vi "电感电阻.vi"() -> ()   [LabVIEW 2017]
panel:
  out "电阻":dbl[](graph)
  out "电感":dbl[](graph)
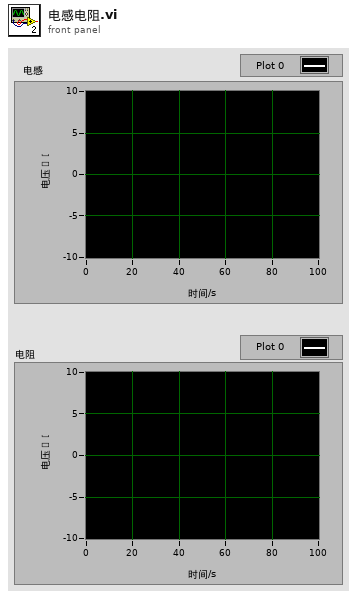
[diagram p1: front panel]
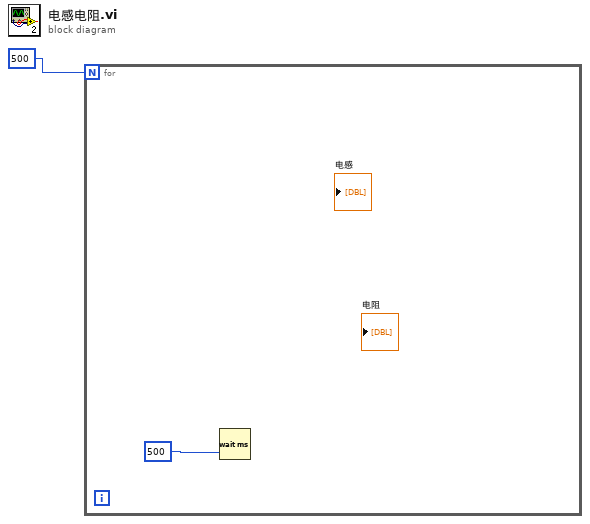
[diagram p0: block diagram]
diagram:
  n1 = for {
    N: 500 -> [_]
    n2 = Wait (ms)(milliseconds to wait=500) -> ()  [unwired: 1 out]
  }
